vi "Add Channel - Right Click.vi"() -> ()   [LabVIEW 2011, in "NI 272x Resistive Simulation Custom Device Configuration.lvlib"]
uses:
  NI 272x Resistive Simulation Custom Device Configuration.lvlib
  <vilib>/NI Veristand/Custom Device API/Custom Device Item Ref.ctl
  <vilib>/NI Veristand/Custom Device API/Custom Device Channel.ctl
  <vilib>/NI Veristand/Custom Device API/Custom Device Channel Type.ctl
  Globals/Names.vi
  <vilib>/NI Veristand/Custom Device API/Set Item Property (I32).vi
  <vilib>/NI Veristand/Custom Device API/Get Item Property (I32).vi
  <vilib>/NI Veristand/Custom Device API/Custom Device API.lvlib
  NI 272x Resistive Simulation Custom Device Shared.lvlib
panel:
  in  "Node Ptr":T1 format="%.0x"
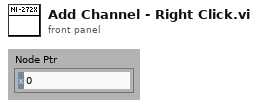
[diagram p1: front panel]
types:
  T1 = typedef "Custom Device API.lvlib/Custom Device Item Ref.ctl" = u64
  T2 = typedef "Custom Device API.lvlib/Custom Device Item Info.ctl" = cluster{"Name":string, "Is Channel":bool, "GUID":string}
  T3 = typedef "Custom Device API.lvlib/Custom Device Channel.ctl" = cluster{"Type":T4, "Units":string, "Default Value":dbl, "Faultable":bool, "Scalable":bool}
  T4 = typedef "Custom Device API.lvlib/Custom Device Channel Type.ctl" = enum16{"Input", "Output"}
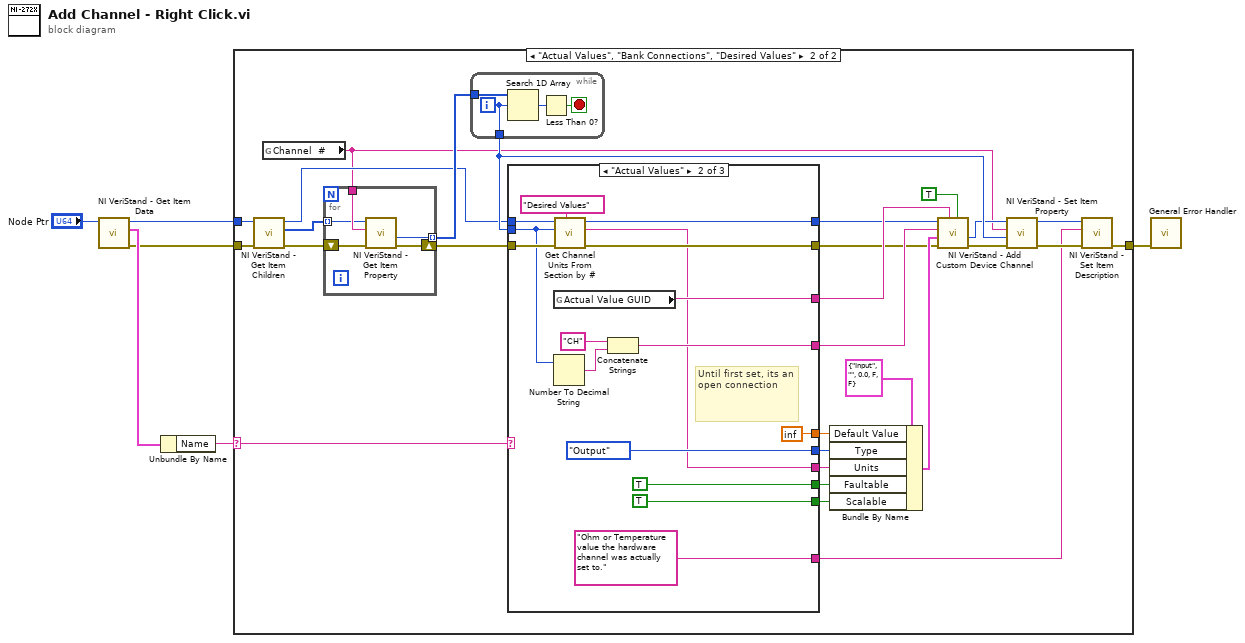
[diagram p0: block diagram]
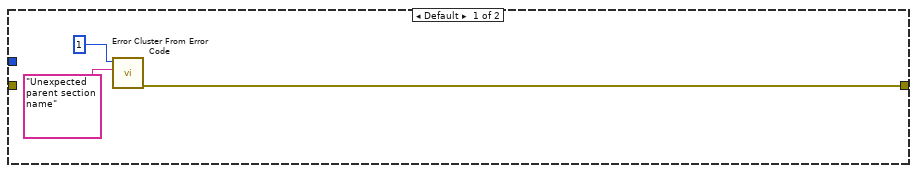
[diagram p2: hidden frame]
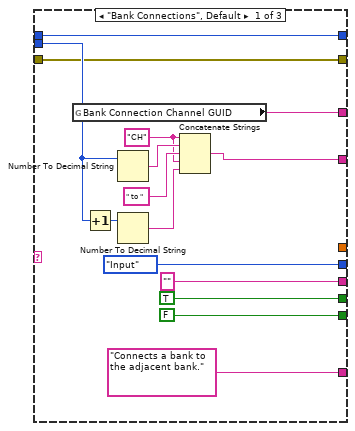
[diagram p3: hidden frame]
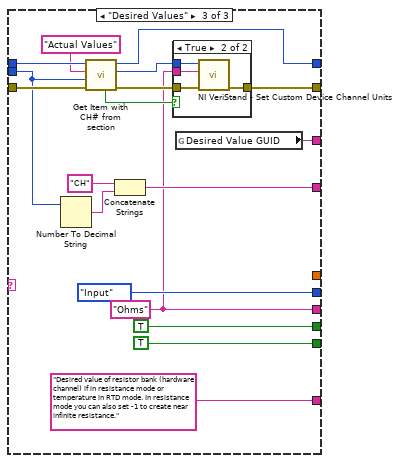
[diagram p4: hidden frame]
diagram:
  n1 = call <vilib>:"NI VeriStand - Get Item Data.vi"("Item Ref in"="Node Ptr") -> ("error out"=w3:errorcluster, "Item Info"=w5:T2, "Item Ref out"=w1:T1)  [unwired: 7 in, 1 out]
  n2 = Unbundle By Name(w5) -> ("Name"=w4:string)
  n3 = case shown="\"Actual Values\", \"Bank Connections\", \"Desired Values\"" w4 {
    selector: w4 -> [_ w31]
    tunnel: w3 -> [_ w37]
    tunnel: [w7 w19] -> w2
    tunnel: w1 -> [_ w36]
    frame Default {
      n4 = call <vilib>:"Error Cluster From Error Code.vi"("error message (\"\")"="Unexpected parent section name" ("error message (\"\")"), "error code (0)"=1) -> ("error out"=w7:errorcluster)  [unwired: 7 in]
    }
    frame "Actual Values", "Bank Connections", "Desired Values" {
      n5 = call <vilib>:"NI VeriStand - Get Item Children.vi"("error in (no error)"=w37, "Item Ref in"=w36) -> ("error out"=w35:errorcluster, "Child Refs"=w34:T1[], "Item Ref out"=w14:T1)  [unwired: 6 in, 1 out]
      n6 = global read "Names.vi" "Channel  #"() -> (w12:string)
      n7 = for {
        shift-right: [w97] -> w15
        shift-left: w35 -> [w100]
        tunnel: w12 -> [w99]
        tunnel: w34 -> [w98] mode=indexing
        tunnel: [w96] -> w33 mode=indexing
        n8 = call-poly <vilib>:"NI VeriStand - Get Item Property.vi"("error in (no error)"=w100, "Property Name"=w99, "Item Ref in"=w98) -> ("error out"=w97:errorcluster, "Value"=w96:i32)  [unwired: 5 in, 2 out]
      }
      n9 = while {
        tunnel: w33 -> [w95]
        tunnel: [w92] -> w23
        i -> [w92]
        stop <- w93 stop-if-true
        n10 = Search 1D Array(1D array=w95, element=w92) -> (index of element=w94:i32)  [unwired: 1 in]
        n11 = Less Than 0?(x=w94) -> (x < 0?=w93:bool)
      }
      n12 = case shown="\"Actual Values\"" w31 {
        tunnel: [Custom_Device_Channel_Type."Input" ("Type") Custom_Device_Channel_Type."Output" ("Type") Custom_Device_Channel_Type."Input" ("Type")] -> w30
        tunnel: ["" ("Units") w54 w70] -> w29
        tunnel: [TRUE ("Faultable") TRUE ("Faultable") TRUE ("Faultable")] -> w28
        tunnel: [FALSE ("Scalable") TRUE ("Scalable") TRUE ("Scalable")] -> w27
        tunnel: w23 -> [w42 w56 w74]
        tunnel: [w43 w63 w81] -> w25
        tunnel: ["Connects a bank to the adjacent bank." "Ohm or Temperature value the hardware channel was actually set to." "Desired value of resistor bank (hardware channel) if in resistance mode or temperature in RTD mode. In resistance mode you can also set -1 to create near infinite resistance."] -> w18
        tunnel: [w40 w61 w79] -> w17
        tunnel: [w39 w59 w73] -> w16
        tunnel: w15 -> [w39 w60 w78]
        tunnel: w14 -> [w38 w58 w77]
        tunnel: [w38 w57 w69] -> w13
        tunnel: [_ inf _] -> w11
        frame "Bank Connections", Default {
          w45 = "CH"
          n13 = global read "Names.vi" "Bank Connection Channel GUID"() -> (w40:string)
          n14 = Increment(x=w42) -> (x+1=w47:i32)
          n15 = Number To Decimal String(number=w42) -> (decimal integer string=w48:string)  [unwired: 1 in]
          n16 = Number To Decimal String(number=w47) -> (decimal integer string=w44:string)  [unwired: 1 in]
          n17 = Concatenate Strings(w45, w48, " to ", w45, w44) -> (w43:string)
        }
        frame "Actual Values" {
          # "Until first set, its an open connection"
          n18 = global read "Names.vi" "Actual Value GUID"() -> (w61:string)
          n19 = Number To Decimal String(number=w56) -> (decimal integer string=w64:string)  [unwired: 1 in]
          n20 = call "Get Channel Units From Section by #.vi"("Section name"="Desired Values", "error in (no error)"=w60, "CH#"=w56, "Item Ref in"=w58) -> ("error out"=w59:errorcluster, "Units"=w54:string, "Item Ref out"=w57:T1)  [unwired: 5 in]
          n21 = Concatenate Strings("CH", w64) -> (w63:string)
        }
        frame "Desired Values" {
          w70 = "Ohms" ("Units")
          n22 = Number To Decimal String(number=w74) -> (decimal integer string=w82:string)  [unwired: 1 in]
          n23 = call "Get Item with CH# from section.vi"("error in (no error)"=w78, "CH#"=w74, "Section containing ch#"="Actual Values" ("Section name"), "Item Ref in"=w77) -> ("error out"=w76:errorcluster, "Matching CH# item in Specified Section"=w71:T1, "Item Ref out"=w69:T1, "Found"=w72:bool)  [unwired: 4 in]
          n24 = Concatenate Strings("CH", w82) -> (w81:string)
          n25 = case shown="True" w72 {
            tunnel: w76 -> [w87 w91]
            tunnel: [w87 w90] -> w73
            tunnel: w71 -> [_ w89]
            tunnel: w70 -> [_ w88]
            frame False {
            }
            frame True {
              n26 = call <vilib>:"NI VeriStand - Set Custom Device Channel Units.vi"("error in (no error)"=w91, "Units"=w88, "Channel Ref in"=w89) -> ("error out"=w90:errorcluster)  [unwired: 7 in, 1 out]
            }
          }
          n27 = global read "Names.vi" "Desired Value GUID"() -> (w79:string)
        }
      }
      n28 = Bundle By Name(cluster=T3 {"Type"=enum."Input", "Units"="", "Default Value"=0.0, "Faultable"=FALSE, "Scalable"=FALSE} ("Channel"), "Default Value"=w11, "Type"=w30, "Units"=w29, "Faultable"=w28, "Scalable"=w27) -> (w26:T3)
      n29 = call <vilib>:"NI VeriStand - Add Custom Device Channel.vi"("Highlight? (F)"=TRUE, "GUID (Default Channel)"=w17, "error in (no error)"=w16, "Channel"=w26, "Channel Name"=w25, "Parent Ref in"=w13) -> ("error out"=w24:errorcluster, "Channel Ref"=w22:T1)  [unwired: 2 in, 2 out]
      n30 = call-poly <vilib>:"NI VeriStand - Set Item Property.vi"("error in (no error)"=w24, "Value"=w23, "Property Name"=w12, "Item Ref in"=w22) -> ("error out"=w20:errorcluster, "Item Ref out"=w21:T1)  [unwired: 5 in, 1 out]
      n31 = call <vilib>:"NI VeriStand - Set Item Description.vi"("error in (no error)"=w20, "Description"=w18, "Item Ref in"=w21) -> ("error out"=w19:errorcluster)  [unwired: 6 in, 2 out]
    }
  }
  n32 = call <vilib>:"General Error Handler.vi"("error in (no error)"=w2) -> ()  [unwired: 10 in, 5 out]
